vi "IP SETTING.vi"() -> ()   [LabVIEW 2017]
uses:
  <vilib>/addons/database/Connection.llb/DB Tools Open Connec (String).vi
  Global/Global 1.vi
  <vilib>/addons/database/NI_Database_API.lvlib
panel:
  in  "SAVE":bool
  in  "Cluster":T1
  out "error out":errorcluster
  in  "error in (no error)":errorcluster
  in  "EXIT":bool
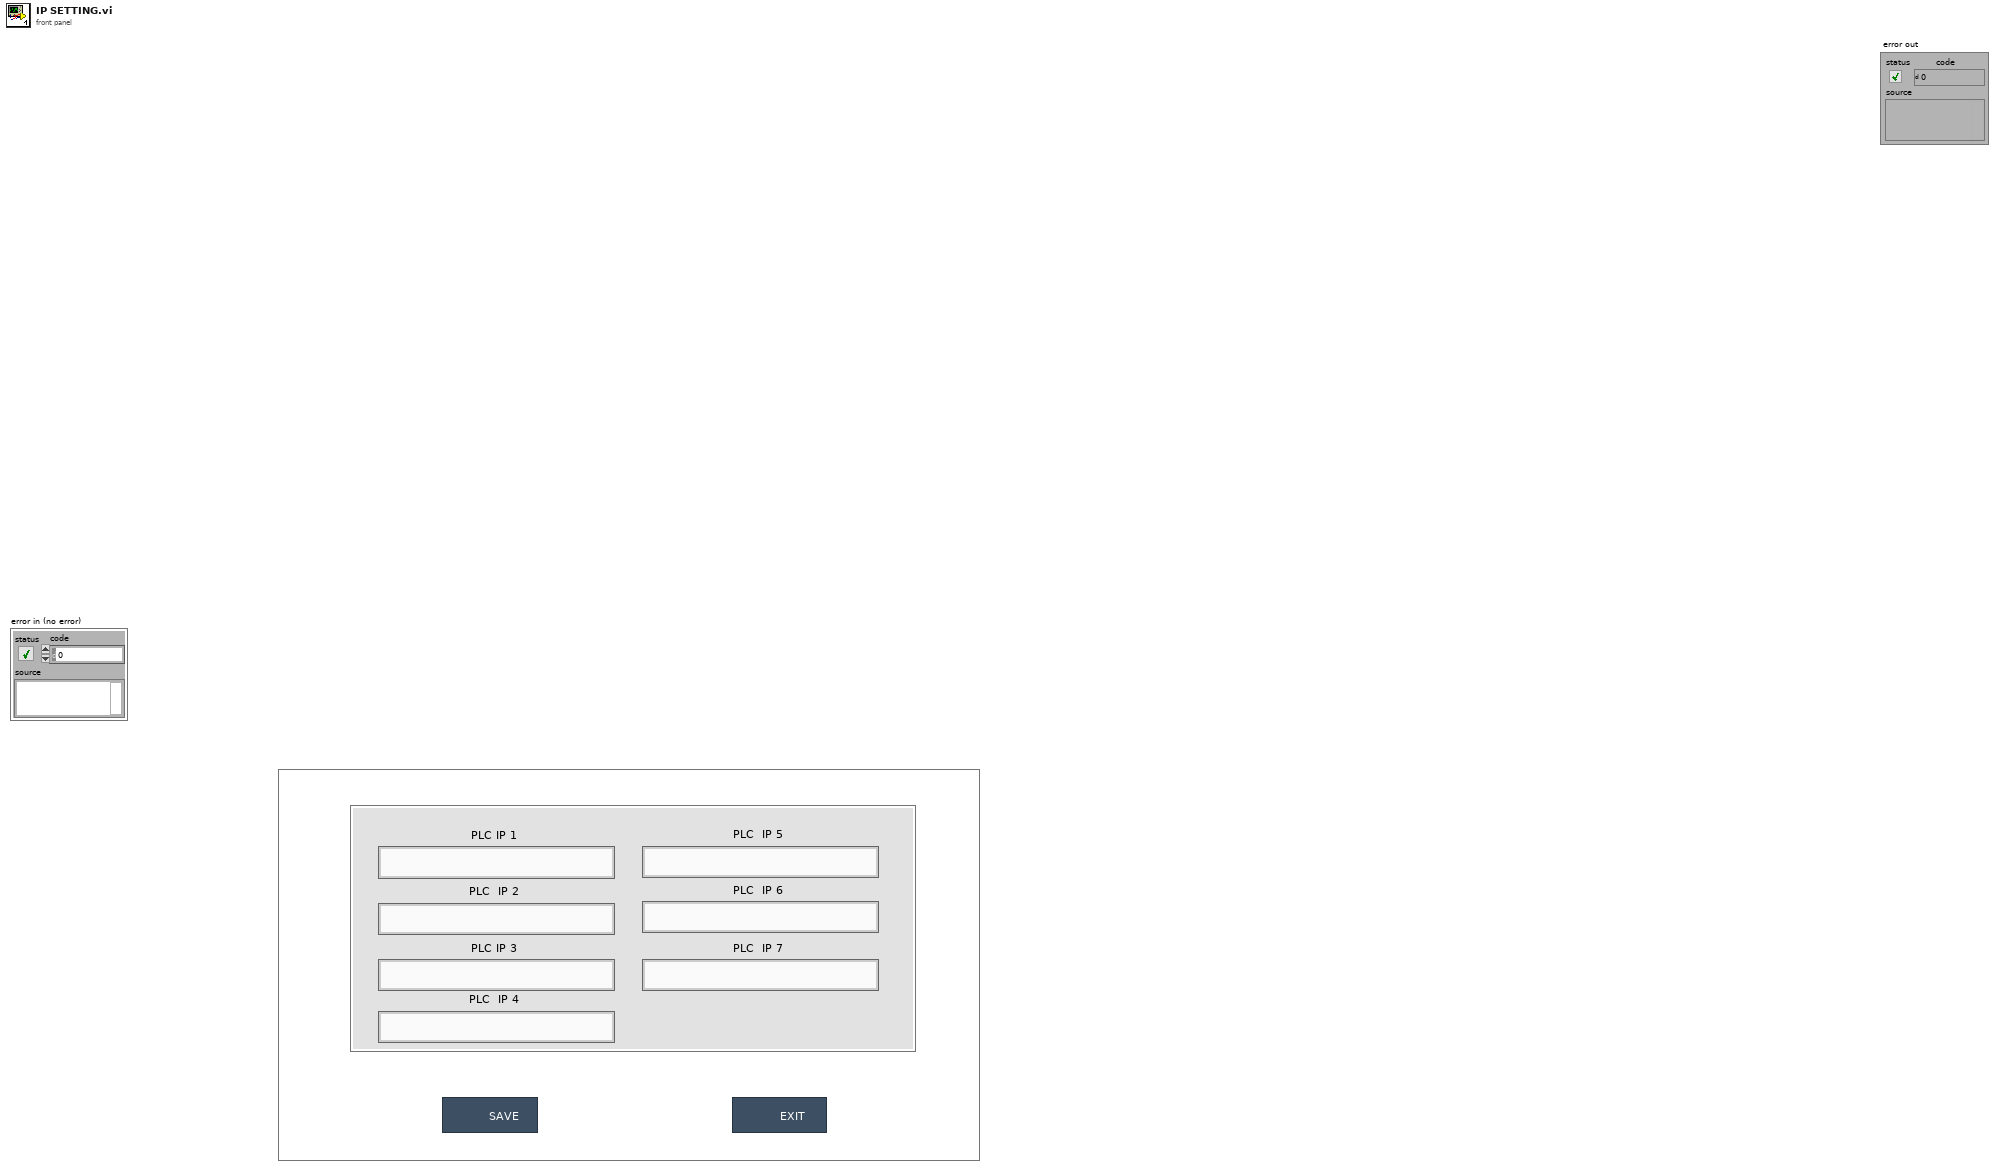
[diagram p1: front panel]
types:
  T1 = cluster{"PLC IP 1":string, "PLC  IP 2":string, "PLC IP 3":string, "PLC  IP 4":string, "PLC  IP 5":string, "PLC  IP 6":string, "PLC  IP 7":string}
  T2 = typedef "NI_Database_API.lvlib/Conn ObjectReference.ctl" = refnum<k1>
  T3 = enum32{"invalid app kind", "Development System", "Run Time System", "Student Edition", "Embedded LabVIEW", "Evaluation", "Custom"}
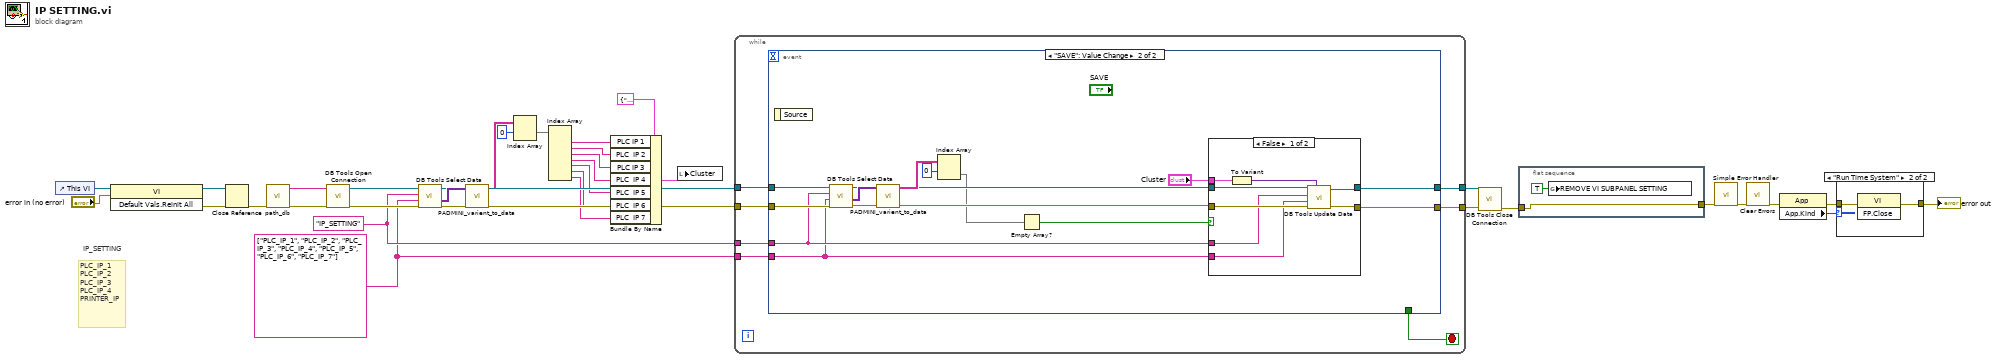
[diagram p0: block diagram]
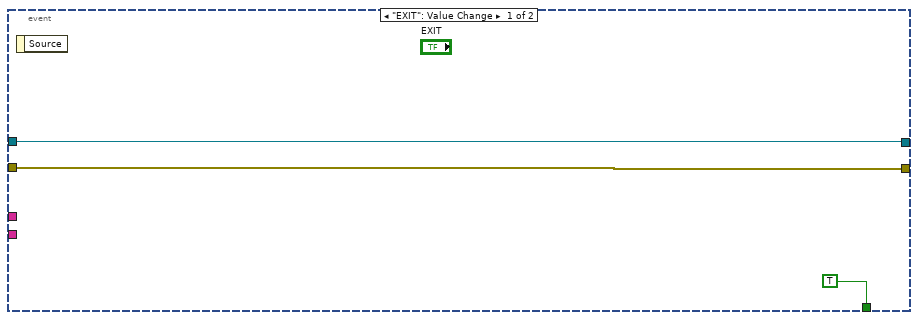
[diagram p2: hidden frame]
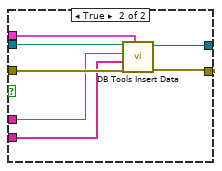
[diagram p3: hidden frame]
diagram:
  w7 = string[] ["PLC_IP_1", "PLC_IP_2", "PLC_IP_3", "PLC_IP_4", "PLC_IP_5", "PLC_IP_6", "PLC_IP_7"] ("columns")
  w12 = "IP_SETTING" ("table")
  # "PLC_IP_1\nPLC_IP_2\nPLC_IP_3\nPLC_IP_4\nPRINTER_IP"
  # "IP_SETTING"
  n1 = control-ref of="This VI"() -> (w36:refnum<vi>)
  n2 = invoke class="VI" method="Default Vals.Reinit All"(reference=w36, error in="error in (no error)") -> (reference out=w34:refnum<vi>, error out=w35:errorcluster)  [unwired: 1 in, 1 out]
  n3 = Close Reference(reference=w34, error in (no error)=w35) -> (error out=w26:errorcluster)
  n4 = call "path_db.vi"("error in"=w26) -> ("error out"=w20:errorcluster, "resulting string"=w25:string)  [unwired: 9 in]
  n5 = call-poly <vilib>:"DB Tools Open Connection.vi"("error in (no error)"=w20, "connection information"=w25) -> ("error out"=w24:errorcluster, "connection reference"=w23:T2)  [unwired: 6 in]
  n6 = call <vilib>:"DB Tools Select Data.vi"("error in (no error)"=w24, "columns"=w7, "table"=w12, "connection reference"=w23) -> ("error out"=w22:errorcluster, "data"=w21:variant[][], "connection reference out"=w15:T2)  [unwired: 2 in]
  n7 = call "PADMINI_varient_to_data.vi"("error in (no error)"=w22, "data"=w21) -> ("error out"=w19:errorcluster, "Array"=w14:string[][])  [unwired: 8 in]
  n8 = Index Array(array=w14, index (row)=0 ("disabled index (col)")) -> (element=w13:string[])  [unwired: 1 in]
  n9 = Index Array(array=w13) -> (element #1=w18:string, element #2=w17:string, element #3=w16:string, element #4=w6:string, element #5=w4:string, element #6=w3:string, element #7=w1:string)  [unwired: 7 in]
  n10 = Bundle By Name(cluster=T1 {"PLC IP 1"="", "PLC  IP 2"="", "PLC IP 3"="", "PLC  IP 4"="", "PLC  IP 5"="", "PLC  IP 6"="", "PLC  IP 7"=""} ("Cluster"), "PLC IP 1"=w18, "PLC  IP 2"=w17, "PLC IP 3"=w16, "PLC  IP 4"=w6, "PLC  IP 5"=w4, "PLC  IP 6"=w3, "PLC  IP 7"=w1) -> (w5:T1)
  n11 = local write "Cluster"(w5) -> ()
  n12 = while {
    tunnel: [w42] -> w10
    tunnel: w19 -> [w43]
    tunnel: w15 -> [w40]
    tunnel: [w39] -> w11
    tunnel: w12 -> [w38]
    tunnel: w7 -> [w37]
    stop <- w41 stop-if-true
    n13 = event shown="[1] \"SAVE\": Value Change" {
      selector: _ -> [_ _]
      dyn-events: _ -> [_ _]
      timeout: _ -> [_ _]
      tunnel: w43 -> [w46 w53]
      tunnel: [w46 w61] -> w42
      tunnel: [TRUE _] -> w41
      tunnel: w40 -> [w44 w54]
      tunnel: [w44 w60] -> w39
      tunnel: w38 -> [_ w52]
      tunnel: w37 -> [_ w51]
      event "EXIT": Value Change {
        n14 = event-data() -> ()  [unwired: 1 in, 1 out]
      }
      event "SAVE": Value Change {
        n15 = event-data() -> ()  [unwired: 1 in, 1 out]
        n16 = call <vilib>:"DB Tools Select Data.vi"("error in (no error)"=w53, "columns"=w51, "table"=w52, "connection reference"=w54) -> ("error out"=w55:errorcluster, "data"=w56:variant[][], "connection reference out"=w49:T2)  [unwired: 2 in]
        n17 = call "PADMINI_varient_to_data.vi"("error in (no error)"=w55, "data"=w56) -> ("error out"=w50:errorcluster, "Array"=w57:string[][])  [unwired: 8 in]
        n18 = Index Array(array=w57, index (row)=0 ("disabled index (col)")) -> (element=w48:string[])  [unwired: 1 in]
        n19 = Empty Array?(array=w48) -> (empty?=w47:bool)
        n20 = case shown="False" w47 {
          tunnel: w50 -> [w68 w76]
          tunnel: w49 -> [w69 w74]
          tunnel: [w66 w75] -> w61
          tunnel: [w67 w73] -> w60
          tunnel: w52 -> [w65 w72]
          tunnel: w51 -> [w64 w71]
          tunnel: "Cluster" -> [w63 w70]
          frame False {
            n21 = To Variant(anything=w63) -> (Variant=w62:variant)
            n22 = call <vilib>:"DB Tools Update Data.vi"("data"=w62, "error in (no error)"=w68, "columns"=w64, "table"=w65, "connection reference"=w69) -> ("error out"=w66:errorcluster, "connection reference out"=w67:T2)  [unwired: 5 in]
          }
          frame True {
            n23 = call <vilib>:"DB Tools Insert Data.vi"("data"=w70, "error in (no error)"=w76, "columns"=w71, "table"=w72, "connection reference"=w74) -> ("error out"=w75:errorcluster, "connection reference out"=w73:T2)  [unwired: 5 in]
          }
        }
      }
    }
  }
  n24 = call <vilib>:"DB Tools Close Connection.vi"("error in (no error)"=w10, "connection reference"=w11) -> ("error out"=w9:errorcluster)  [unwired: 5 in]
  n25 = flat-sequence {
    tunnel: w9 -> [w78]
    tunnel: [w78] -> w27
    frame #0 {
      n26 = global write "Global 1.vi" "REMOVE VI SUBPANEL SETTING"(TRUE ("REMOVE_VI _SUBPANEL_3")) -> ()
    }
  }
  n27 = call <vilib>:"Simple Error Handler.vi"("error in (no error)"=w27) -> ("error out"=w32:errorcluster)  [unwired: 4 in, 4 out]
  n28 = call <vilib>:"Clear Errors.vi"("error in (no error)"=w32) -> ("error out"=w29:errorcluster)  [unwired: 5 in, 1 out]
  n29 = property class="App"(error in=w29) -> (error out=w30:errorcluster, "App.Kind"=w31:T3)  [unwired: 1 in, 1 out]
  n30 = case shown="\"Run Time System\"" w31 {
    tunnel: w30 -> [w79 w81]
    tunnel: [w79 w80] -> w28
    frame Default {
    }
    frame "Run Time System" {
      n31 = invoke class="VI" method="FP.Close"(error in=w81) -> (error out=w80:errorcluster)  [unwired: 2 in, 2 out]
    }
  }
  "error out" <- w28
